vi "Integrate Stop.vi"(8 "error in (no error)":errorcluster, 10 "Element (True)":bool[](array[boolean])=[TRUE, TRUE, TRUE, TRUE, TRUE, TRUE], 11 "VISA resource name":refnum<visa-resource-name>) -> (0 "error out":errorcluster, 3 "VISA resource name out":refnum<visa-resource-name>)   [LabVIEW 2021, in "Yokogawa WT1800 Series.lvlib"]
doc: "Stops integration."
uses:
  <instrlib>/Yokogawa WT1800 Series/Yokogawa WT1800 Series.lvlib
panel:
  # "Element 1"
  # "Element 2"
  # "Element 3"
  # "Element 4"
  # "Element 5"
  # "Element 6"
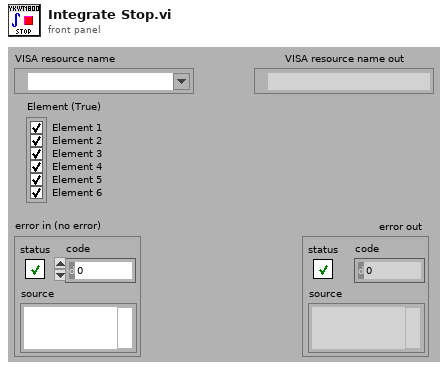
[diagram p1: front panel]
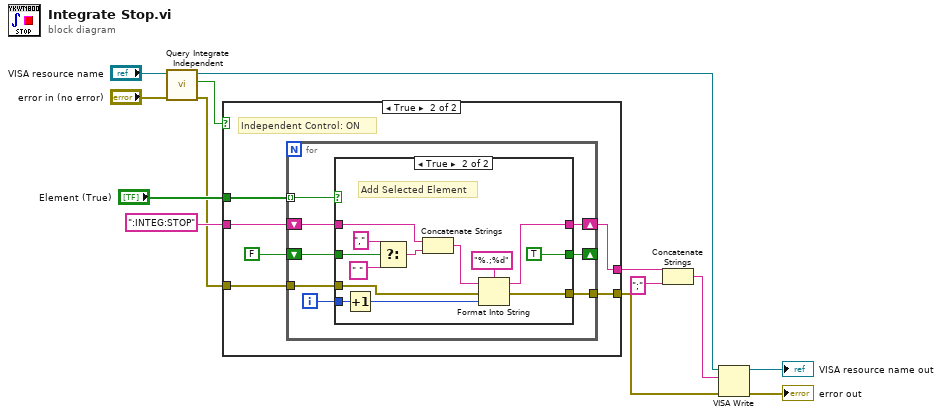
[diagram p0: block diagram]
diagram:
  n1 = call <instrlib>:"Query Integrate Independent.vi"("error in (no error)"="error in (no error)", "VISA resource name"="VISA resource name") -> ("error out"=w2:errorcluster, "Independent Control"=w8:bool, "VISA resource name out"=w10:refnum<visa-resource-name>)  [unwired: 7 in]
  n2 = case shown="True" w8 {
    tunnel: ":INTEG:STOP" -> [w15 w19]
    tunnel: [w15 w16] -> w4
    tunnel: "Element (True)" -> [_ w21]
    tunnel: w2 -> [w14 w18]
    tunnel: [w14 w17] -> w1
    frame False {
      # "Independent Control: OFF"
    }
    frame True {
      # "Independent Control: ON"
      n3 = for {
        tunnel: w21 -> [w27] mode=indexing
        shift-right: [w26] -> _
        shift-left: FALSE -> [w29]
        tunnel: w18 -> [w24]
        tunnel: [w23] -> w17
        shift-right: [w22] -> w16
        shift-left: w19 -> [w28]
        i -> [w25]
        n4 = case shown="True" w27 {
          tunnel: w29 -> [w32 w45]
          tunnel: w28 -> [w30 w42]
          tunnel: [w32 TRUE] -> w26
          tunnel: w25 -> [_ w40]
          tunnel: w24 -> [w31 w36]
          tunnel: [w31 w35] -> w23
          tunnel: [w30 w34] -> w22
          frame False {
            # "Element not selected"
          }
          frame True {
            # "Add Selected Element"
            n5 = Increment(x=w40) -> (x+1=w39:i32)
            n6 = Select(t="," ("文字列"), s=w45, f=" " ("文字列")) -> (s? t:f=w41:string)
            n7 = Concatenate Strings(w42, w41) -> (w38:string)
            n8 = Format Into String(format string="%.;%d" ("形式文字列"), initial string=w38, error in=w36, w39) -> (resulting string=w34:string, error out=w35:errorcluster)
          }
        }
      }
    }
  }
  n9 = Concatenate Strings(w4, ";" ("文字列")) -> (w3:string)
  n10 = VISA Write ("VISA書き込み")(VISA resource name=w10, write buffer=w3, error in (no error)=w1) -> (VISA resource name out=→"VISA resource name out":refnum<visa-resource-name>, error out=→"error out":errorcluster)  [unwired: 1 out]
